vi "mod_VSB filter design.vi"(0 "VSB FIR filter design":T1={"#taps"=161, "lower PB (Hz)"=-0.0375, "upper PB (Hz)"=0.2, "lower SB (Hz)"=-0.0625, "upper SB (Hz)"=0.225} {"lower SB (Hz)" format="%0.2p"; "upper SB (Hz)" format="%0.2p"; "lower PB (Hz)" format="%0.2p"; "upper PB (Hz)" format="%0.2p"}, 11 "error in (no error)":errorcluster, 13 "reset ? (T)":bool=TRUE) -> (4 "VSB filter taps":cdb[](array[numeric]), 15 "error out":errorcluster)   [LabVIEW 2020, in "niAMT.lvlib"]
uses:
  <vilib>/addons/Modulation/niAMT.lvlib
  <vilib>/addons/Modulation/Analog/controls/mod_AM VSB filter.ctl
  <vilib>/Analysis/2dsp.llb/1D Convolution (DBL).vi
  <vilib>/measure/NI_MAPro.lvlib
  <vilib>/Analysis/NI_AALPro.lvlib
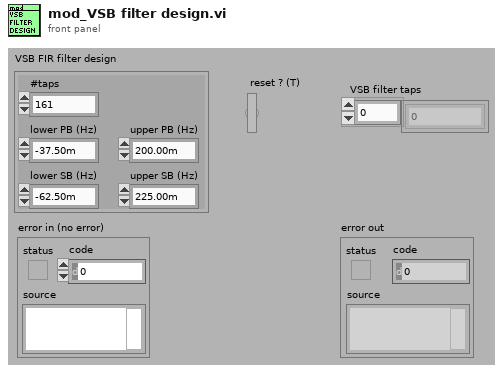
[diagram p1: front panel]
types:
  T1 = typedef "niAMT.lvlib/mod_AM VSB filter.ctl" = cluster{"#taps":i32, "lower PB (Hz)":dbl, "upper PB (Hz)":dbl, "lower SB (Hz)":dbl, "upper SB (Hz)":dbl}
  T2 = cluster{"Topology":enum16{"Off", "FIR by Specification", "Equi-ripple FIR", "Windowed FIR"}, "Type":enum16{"Lowpass", "Highpass", "Bandpass", "Bandstop"}, "#Taps":i32, "Lower PB":dbl, "Upper PB":dbl, "Lower SB":dbl, "Upper SB":dbl}
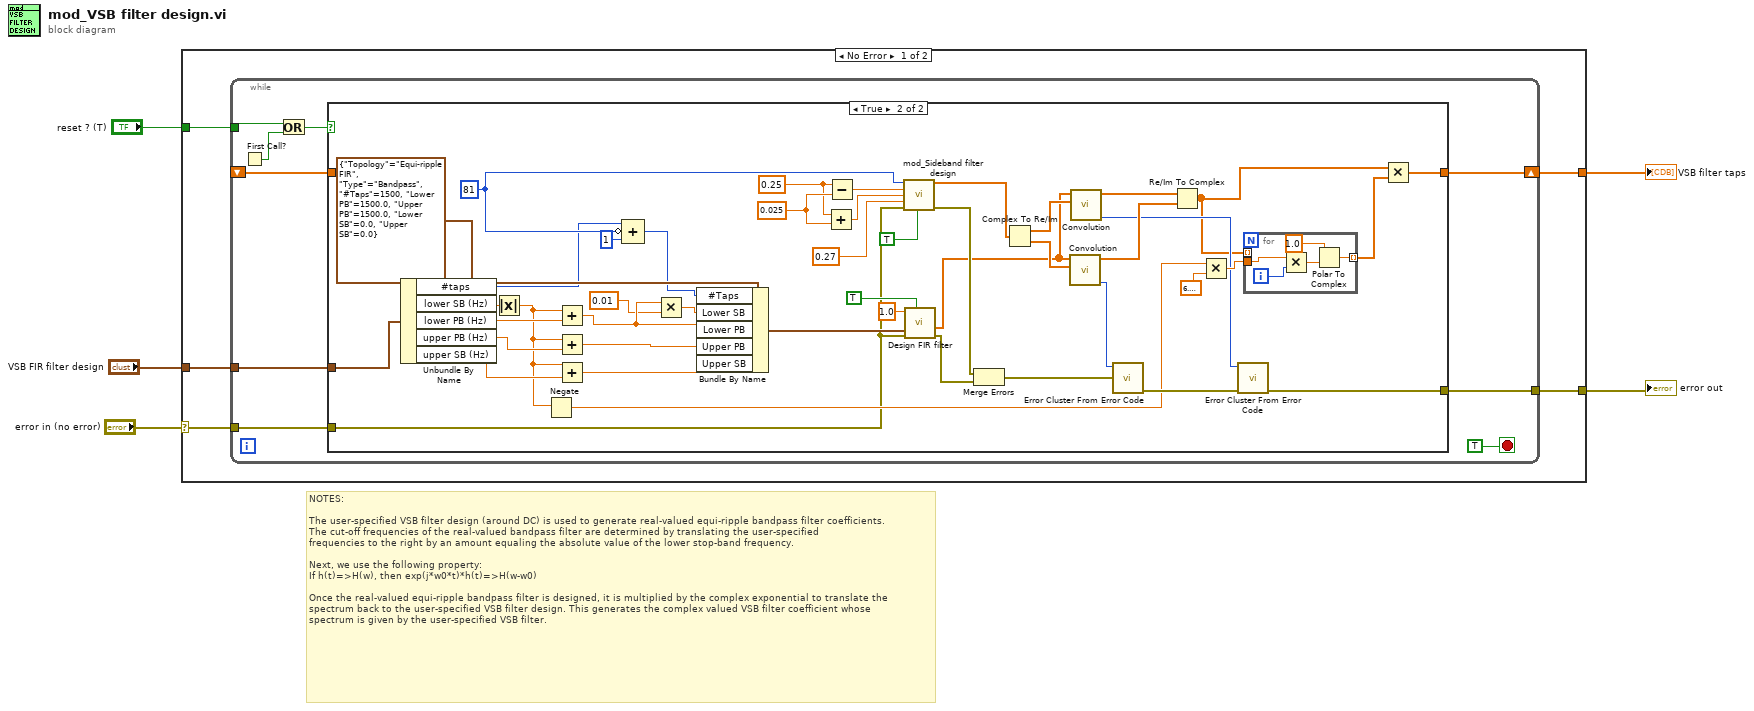
[diagram p0: block diagram]
diagram:
  # "NOTES:\n\nThe user-specified VSB filter design (around DC) is used to generate real-valued equi-ripple bandpass filter coefficients.\nThe cut-off frequencies of the real-valued bandpass filter are determined by translating the user-specified\nfrequencies to the right by an amount equaling the absolute value of the lower stop-band frequency.\n\nNext, we use the following property: \nIf h(t)=>H(w), then exp(j*w0*t)*h(t)=>H(w-w0)\n\nOnce the real-valued equi-ripple bandpass filter is designed, it is multiplied by the complex exponential to translate the\nspectrum back to the user-specified VSB filter design. This generates the complex valued VSB filter coefficient whose\nspectrum is given by the user-specified VSB filter."
  n1 = case shown="No Error" "error in (no error)" {
    selector: "error in (no error)" -> [w10 w72]
    tunnel: [w9 w72] -> w4
    tunnel: "VSB FIR filter design" -> [w8 _]
    tunnel: "reset ? (T)" -> [w7 _]
    tunnel: [w6 _] -> w1
    frame No Error {
      n2 = while {
        tunnel: w7 -> [w12]
        shift-right: [w19] -> w6
        shift-left: _ -> [w17]
        tunnel: w10 -> [w16]
        tunnel: [w15] -> w9
        tunnel: w8 -> [w14]
        stop <- TRUE stop-if-true
        n3 = First Call?() -> (First Call?: T/F=w13:bool)
        n4 = Or(x=w12, y=w13) -> (x .or. y?=w11:bool)
        n5 = case shown="True" w11 {
          tunnel: [w21 w66] -> w19
          tunnel: w17 -> [w21 _]
          tunnel: w16 -> [w20 w26]
          tunnel: [w20 w55] -> w15
          tunnel: w14 -> [_ w51]
          frame False {
          }
          frame True {
            w32 = 0.025 ("center frequency")
            w31 = 0.25 ("center frequency")
            w34 = 81 ("Taps")
            n6 = Unbundle By Name(w51) -> ("#taps"=w22:i32, "lower SB (Hz)"=w48:dbl, "lower PB (Hz)"=w47:dbl, "upper PB (Hz)"=w46:dbl, "upper SB (Hz)"=w45:dbl)
            n7 = Absolute Value(x=w48) -> (abs(x)=w41:dbl)
            n8 = Negate(x=w41) -> (-x=w40:dbl)
            n9 = Add(x=w41, y=w47) -> (x+y=w39:dbl)
            n10 = Add(x=w41, y=w46) -> (x+y=w44:dbl)
            n11 = Add(x=w41, y=w45) -> (x+y=w43:dbl)
            n12 = Compound Arithmetic op=ADD(w22, invert w34, 1 ("value")) -> (w36:i32)
            n13 = Multiply(x=w39, y=0.01) -> (x*y=w37:dbl)
            n14 = Bundle By Name(cluster=T2 {"Topology"=enum."Equi-ripple FIR", "Type"=enum."Bandpass", "#Taps"=1500, "Lower PB"=1500.0, "Upper PB"=1500.0, "Lower SB"=0.0, "Upper SB"=0.0} ("FIR filter specifications"), "#Taps"=w36, "Lower SB"=w37, "Lower PB"=w39, "Upper PB"=w44, "Upper SB"=w43) -> (w42:T2)
            n15 = Add(x=w31, y=w32) -> (x+y=w30:dbl)
            n16 = Subtract(x=w31, y=w32) -> (x-y=w33:dbl)
            n17 = call <vilib>:"mod_Sideband filter design.vi"("taps"=w34, "lower pass band frequency"=w33, "lower stop band frequency"=w30, "frequency shift"=0.27, "error in (no error)"=w26, "reset? (T)"=TRUE ("reset")) -> ("filter taps"=w28:cdb[], "error out"=w27:errorcluster)  [unwired: 8 out]
            n18 = call <vilib>:"Design FIR filter.vi"("FIR filter specifications"=w42, "redesign filter"=TRUE ("reset"), "error in"=w26, "dt"=1.0) -> ("error out"=w52:errorcluster, "forward coefficients"=w23:dbl[])  [unwired: 3 in, 3 out]
            n19 = Merge Errors(w27, w52) -> (w54:errorcluster)
            n20 = Complex To Re/Im(x + iy=w28) -> (x=w62:dbl[], y=w61:dbl[])
            n21 = call-poly <vilib>:"Convolution.vi"("Y"=w61, "X"=w23) -> ("error"=w57:i32, "X * Y"=w59:dbl[])  [unwired: 1 in, 7 out]
            n22 = call-poly <vilib>:"Convolution.vi"("Y"=w62, "X"=w23) -> ("error"=w58:i32, "X * Y"=w60:dbl[])  [unwired: 1 in, 7 out]
            n23 = call <vilib>:"Error Cluster From Error Code.vi"("error in (no error)"=w54, "error code (0)"=w57) -> ("error out"=w56:errorcluster)  [unwired: 1 in, 6 out]
            n24 = Re/Im To Complex(1:w59, 2:w60) -> (0:w35:cdb[])
            n25 = Multiply(x=w40, y=6.283185307179586) -> (x*y=w64:dbl)
            n26 = call <vilib>:"Error Cluster From Error Code.vi"("error in (no error)"=w56, "error code (0)"=w58) -> ("error out"=w55:errorcluster)  [unwired: 1 in, 6 out]
            n27 = for {
              tunnel: [w68] -> w63 mode=indexing
              tunnel: w64 -> [w67]
              tunnel: w35 -> [_] mode=indexing
              i -> [w71]
              n28 = Multiply(x=w67, y=w71) -> (x*y=w70:dbl)
              n29 = Polar To Complex(1:w70, 2:1.0 ("r")) -> (0:w68:cdb)
            }
            n30 = Multiply(x=w35, y=w63) -> (x*y=w66:cdb[])
          }
        }
      }
    }
    frame Error {
    }
  }
  "error out" <- w4
  "VSB filter taps" <- w1
